vi "scriptRunner.vi"(8 "error in (no error)":errorcluster, 9 "script":string, 10 "matlabScript":string, 11 "MatlabScripts in":refnum<class "MatlabScripts.lvclass">) -> (0 "error out":errorcluster, 3 "MatlabScripts out":refnum<class "MatlabScripts.lvclass">)   [LabVIEW 2009, in "Views.lvlib" / "ExperimentControl.lvlib" / "MatlabScripts.lvclass"]
uses:
  MatlabScripts.lvclass
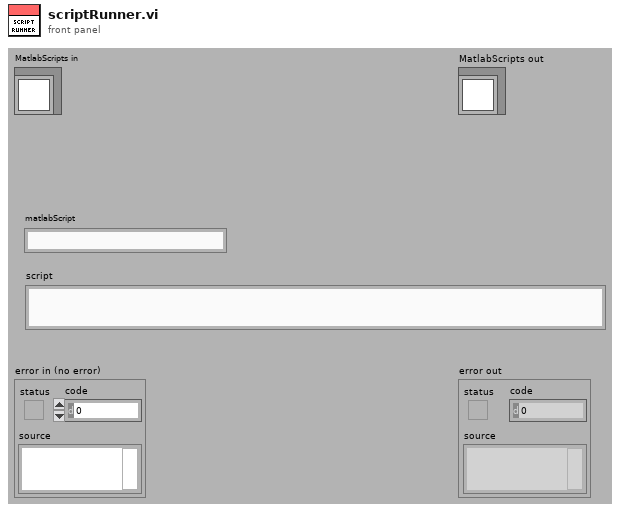
[diagram p1: front panel]
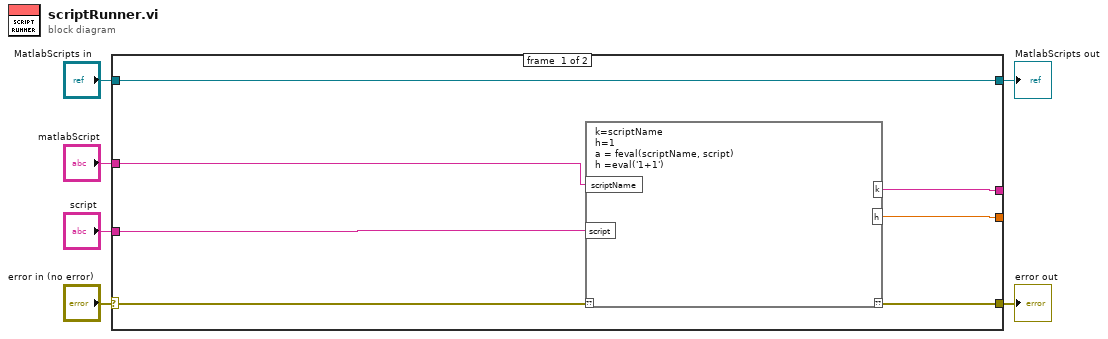
[diagram p0: block diagram]
diagram:
  n1 = case shown="No Error" "error in (no error)" {
    selector: "error in (no error)" -> [w12 w15]
    tunnel: [w11 w15] -> w5
    tunnel: [w13 w14] -> w3
    tunnel: "MatlabScripts in" -> [w13 w14]
    tunnel: "matlabScript" -> [w9 _]
    tunnel: "script" -> [w10 _]
    tunnel: [w8 _] -> _
    tunnel: [w7 _] -> _
    frame #0 {
      n2 = script code="k=scriptName\nh=1\na = feval(scriptName, script)\nh =eval('1+1')"("??"=w12, "scriptName"=w9, "script"=w10) -> ("??"=w11:errorcluster, "k"=w8:string, "h"=w7:dbl)
    }
    frame #1 {
    }
  }
  "error out" <- w5
  "MatlabScripts out" <- w3
